vi "PWM.vi"() -> ()   [LabVIEW 2014]
doc: "This example demonstrates how to generate digital output data using software timing.\n\nFor instructions on how to connect your signals from the DAQ device, refer to your device documentation."
uses:
  <vilib>/Utility/error.llb/DialogType.ctl
  <vilib>/DAQmx/write.llb/DAQmx Write (Digital Bool 1Line 1Point).vi
  <vilib>/DAQmx/create/channels.llb/DAQmx Create Channel (DO-Digital Output).vi
  <vilib>/DAQmx/miscellaneous.llb/DAQmx Fill In Error Info.vi
panel:
  in  "Loop time":u32
  in  "On Time":u32
  in  "Stop":bool
  in  "Line(s)":tag="Dev1/port0/line0:1"
  # "Channel Settings"
  # "Channel Settings"
  # "Timing Settings"
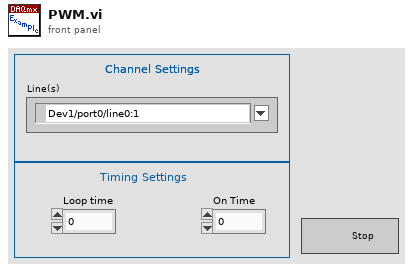
[diagram p1: front panel]
types:
  T1 = typedef "DialogType.ctl" = u16
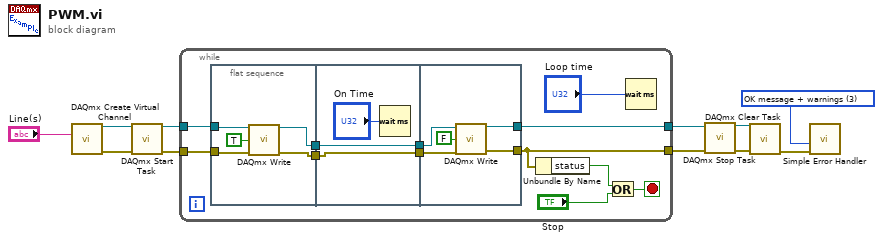
[diagram p0: block diagram]
diagram:
  w3 = T1 3 items=["no dialog", "OK message", "continue or stop message", "OK message + warnings", "continue/stop + warnings"] ("type of dialog (OK msg:1)")
  n1 = call-poly <vilib>:"DAQmx Create Virtual Channel.vi"("lines"="Line(s)") -> ("task out"=w6:refnum<k21>, "error out"=w7:errorcluster)  [unwired: 13 in]
  n2 = call <vilib>:"DAQmx Start Task.vi"("task/channels in"=w6, "error in"=w7) -> ("task out"=w11:refnum<k21>, "error out"=w10:errorcluster)  [unwired: 12 in]
  n3 = while {
    tunnel: w11 -> [w23]
    tunnel: w10 -> [w22]
    tunnel: [w13] -> w2
    tunnel: [w12] -> w1
    stop <- w21 stop-if-true
    n4 = flat-sequence {
      tunnel: w23 -> [w27]
      tunnel: w22 -> [w26]
      tunnel: [w25] -> w16
      tunnel: [w24] -> w14
      tunnel: [w30] -> w17
      tunnel: w16 -> [w30]
      tunnel: [w29] -> w15
      tunnel: w14 -> [w29]
      tunnel: w17 -> [w36]
      tunnel: w15 -> [w35]
      tunnel: [w34] -> w13
      tunnel: [w33] -> w12
      frame #0 {
        n5 = call-poly <vilib>:"DAQmx Write.vi"("task/channels in"=w27, "data"=TRUE, "error in"=w26) -> ("task out"=w25:refnum<k21>, "error out"=w24:errorcluster)  [unwired: 10 in, 1 out]
      }
      frame #1 {
        n6 = Wait (ms)(milliseconds to wait="On Time") -> ()  [unwired: 1 out]
      }
      frame #2 {
        n7 = call-poly <vilib>:"DAQmx Write.vi"("task/channels in"=w36, "data"=FALSE, "error in"=w35) -> ("task out"=w34:refnum<k21>, "error out"=w33:errorcluster)  [unwired: 10 in, 1 out]
      }
    }
    n8 = Unbundle By Name(w12) -> ("status"=w20:bool)
    n9 = Or(x=w20, y="Stop") -> (x .or. y?=w21:bool)
    n10 = Wait (ms)(milliseconds to wait="Loop time") -> ()  [unwired: 1 out]
  }
  n11 = call <vilib>:"DAQmx Stop Task.vi"("task/channels in"=w2, "error in"=w1) -> ("task out"=w5:refnum<k21>, "error out"=w4:errorcluster)  [unwired: 12 in]
  n12 = call <vilib>:"DAQmx Clear Task.vi"("task in"=w5, "error in"=w4) -> ("error out"=w9:errorcluster)  [unwired: 13 in]
  n13 = call <vilib>:"Simple Error Handler.vi"("type of dialog (OK msg:1)"=w3, "error in (no error)"=w9) -> ()  [unwired: 3 in, 5 out]
